vi "Configure.vi"(8 "error in (no error)":errorcluster) -> (0 "error out":errorcluster, 2 "valid config":bool, 3 "config":T1)   [LabVIEW 2017, in "IrDataEventCreator.lvlib"]
uses:
  <vilib>/addons/InsightCM/Devices/Shared/Ir/IrDataEventCreator/IrDataEventCreator.lvlib
  <vilib>/addons/InsightCM/Devices/Shared/Ir/IrDataEventCreator/controls/config.ctl
  <vilib>/addons/InsightCM/Utilities/GlobalConfiguration/GlobalConfiguration.lvlib
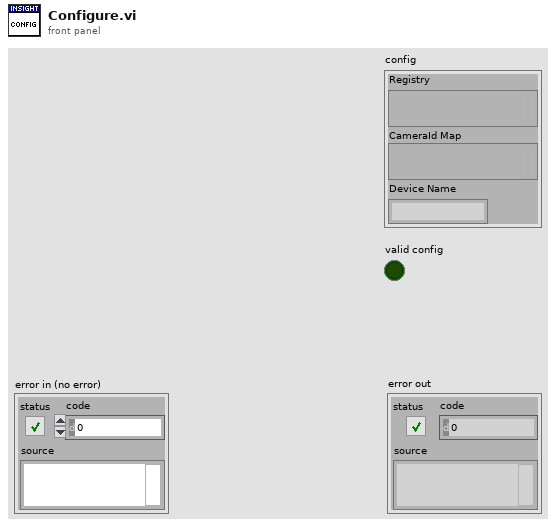
[diagram p1: front panel]
types:
  T1 = typedef "IrDataEventCreator.lvlib/config.ctl" = cluster{"Registry":variant, "CameraId Map":variant, "Device Name":string}
  T2 = typedef "R2_Device.ctl" = cluster{"Id":string, "Name":string, "DeviceType":string, "HardwareName":string, "IpAddress":string, "HardwareInfo":T3[], "ApplicationType":string, "ApplicationVersion":string, "EquipmentIds":string[], "ConfigurationVersion":string, "State":T4, "Properties":T3[], "DataGroups":T5[], "BurstModeTrigger":T9, "SensorGroups":T10[]}
  T3 = typedef "KeyValuePair.ctl" = cluster{"Key":string, "Value":string}
  T4 = typedef "DeviceState.ctl" = cluster{"Disabled":bool}
  T5 = typedef "R2_DataGroup.ctl" = cluster{"Name":string, "OperatingStates":T6[], "Properties":T3[], "EquipmentIds":string[], "AssetNodeId":string}
  T6 = typedef "OperatingState.ctl" = cluster{"Name":string, "Properties":T3[], "Triggers":T7[]}
  T7 = typedef "Trigger.ctl" = cluster{"Type":string, "Expression":string, "Conditions":T8[]}
  T8 = typedef "Condition.ctl" = cluster{"Source":string, "Type":string, "Operator":string, "CompareTo":string, "DwellSeconds":dbl}
  T9 = typedef "BurstModeTrigger.ctl" = cluster{"Trigger":T7, "SampleRate":string, "AcquisitionLength":string}
  T10 = typedef "DeviceSensorGroup.ctl" = cluster{"EquipId":string, "SensorGroupId":string, "Endpoints":T11[]}
  T11 = typedef "Endpoint.ctl" = cluster{"Type":string, "Address":string, "Properties":T3[], "Channels":T12[]}
  T12 = typedef "WirelessChannel.ctl" = cluster{"ChannelNumber":i32, "AssetId":string}
  T13 = typedef "Camera.ctl" = cluster{"Id":string, "Name":string, "Properties":T3[], "Triggers":T7[]}
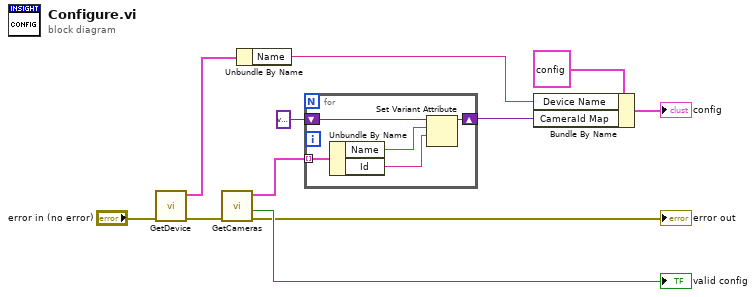
[diagram p0: block diagram]
diagram:
  n1 = call <vilib>:"GetDevice.vi"("error in (no error)"="error in (no error)") -> ("error out"=w3:errorcluster, "device configuration"=w2:T2)  [unwired: 8 in, 1 out]
  n2 = call <vilib>:"GetCameras.vi"("error in (no error)"=w3) -> ("error out"=→"error out":errorcluster, "found"=→"valid config":bool, "cameras"=w7:T13[])  [unwired: 8 in]
  n3 = Unbundle By Name(w2) -> ("Name"=w1:string)
  n4 = for {
    shift-right: [w14] -> w8
    shift-left: variant -> [w15]
    tunnel: w7 -> [w16] mode=indexing
    n5 = Unbundle By Name(w16) -> ("Name"=w13:string, "Id"=w12:string)
    n6 = Set Variant Attribute(Variant=w15, name=w13, value=w12) -> (Variant out=w14:variant)  [unwired: 1 in, 2 out]
  }
  n7 = Bundle By Name(cluster=T1 {"Registry"=variant, "CameraId Map"=variant, "Device Name"=""} ("config 2"), "Device Name"=w1, "CameraId Map"=w8) -> (→"config":T1)
